vi "S7 TCP Test.vi"() -> ()   [LabVIEW 2017]
uses:
  S7 TCP API Library/S7 TCP.lvlib
panel:
  out "error out 2":errorcluster
  in  "milliseconds to wait":u32=1000
  in  "IP Address":string="10.0.0.5"
  in  "Data Block #":u16=1
  out "Loop Itteration":i32
  in  "Stop":bool
  out "Data Element 0 as Boolean array":bool[](array[boolean])
  in  "Read / Write":u8(ring)=4 items=["Read"=4, "Write"=5]
  in  "Address Areas":u8(ring)=131 items=["I/O (P)"=128, "Input (I)"=129, "Output (Q)"=130, "Bit Memory (M)"=131, "Data (DB)"=132, "Instance Data (DI)"=133, "Local Data (L)"=134, "Predecessor Local Data (VL)"=135]
  in  "Start Address (bytes)":u32
  out "Read Data":u8[](array[numeric]) format="%.0x"
  in  "Read Length (bytes)":u16=1
  in  "Write Data":i32
  out "Data Valid":bool
  out "error out":errorcluster
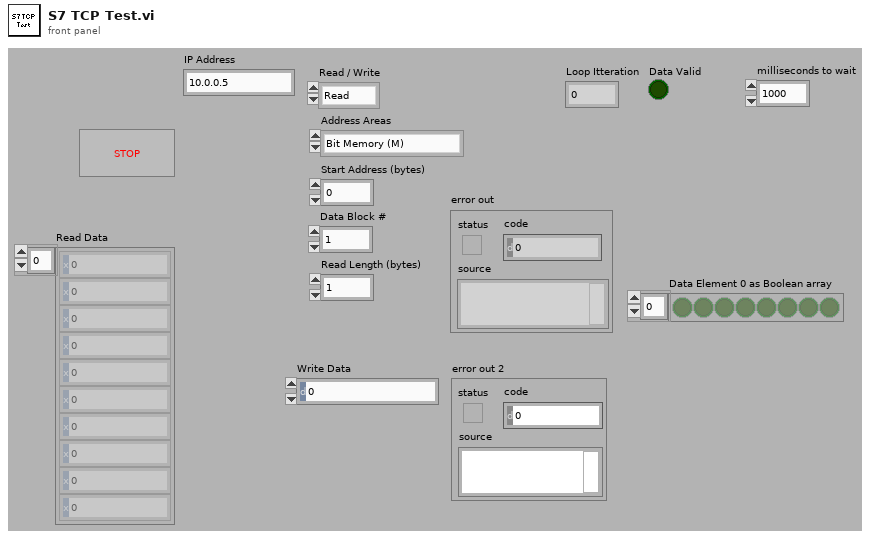
[diagram p1: front panel]
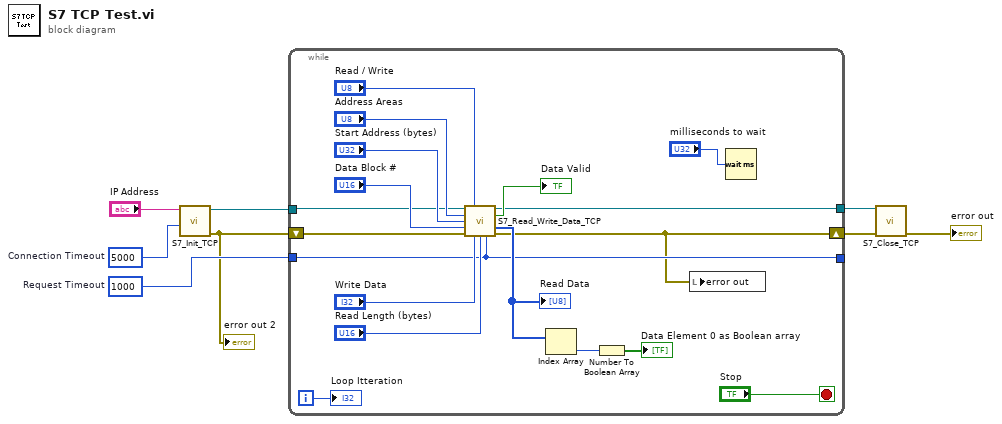
[diagram p0: block diagram]
diagram:
  w6 = u32 1000  # Request Timeout
  w7 = u32 5000  # Connection Timeout
  n1 = call "S7_Init_TCP.vi"("Connection Timeout"=w7, "IP Address"="IP Address") -> ("error out"=w3:errorcluster, "TCP Connection Ref"=w4:refnum<k5>)  [unwired: 3 in, 5 out]
  "error out 2" <- w3
  n2 = while {
    tunnel: w4 -> [w10]
    tunnel: w6 -> [w14]
    tunnel: [w14] -> _
    shift-right: [w11] -> w5
    shift-left: w3 -> [w21]
    tunnel: [w9] -> w1
    i -> [w15]
    stop <- "Stop" stop-if-true
    n3 = call "S7_Read_Write_Data_TCP.vi"("TCP Connection Ref"=w10, "Read / Write"="Read / Write", "Address Areas"="Address Areas", "Start Address (bytes)"="Start Address (bytes)", "Data Block #"="Data Block #", "error in"=w21, "Write Data"="Write Data", "Length (bytes)"="Read Length (bytes)", "Timeout"=w14) -> ("TCP Connection Ref Out"=w9:refnum<k5>, "Data Valid"=→"Data Valid":bool, "Data Read"=w20:u8[], "error out"=w11:errorcluster)  [unwired: 1 in, 2 out]
    "Read Data" <- w20
    n4 = Index Array(array=w20) -> (element=w19:u8)  [unwired: 1 in]
    n5 = Number To Boolean Array(number=w19) -> (Boolean array=→"Data Element 0 as Boolean array":bool[])
    n6 = local write "error out"(w11) -> ()
    n7 = Wait (ms)(milliseconds to wait="milliseconds to wait") -> ()  [unwired: 1 out]
    "Loop Itteration" <- w15
  }
  n8 = call "S7_Close_TCP.vi"("error in"=w5, "TCP Connection Ref"=w1) -> ("error out"=→"error out":errorcluster)  [unwired: 1 in, 8 out]
